vi "Remove Device.vi"(8 "error in (no error)":errorcluster, 11 "Configuration Editor in":refnum<class "Configuration Editor.lvclass">) -> (0 "error out":errorcluster, 3 "Configuration Editor out":refnum<class "Configuration Editor.lvclass">)   [LabVIEW 2023, in "Configuration Editor.lvlib" / "Configuration Editor.lvclass"]
uses:
  Library/Configuration Editor.lvclass
  Library/Configuration Editor.lvclass/Configuration Editor.ctl
  builds/Framework/Configuration.lvlibp/Library/Configuration.lvclass
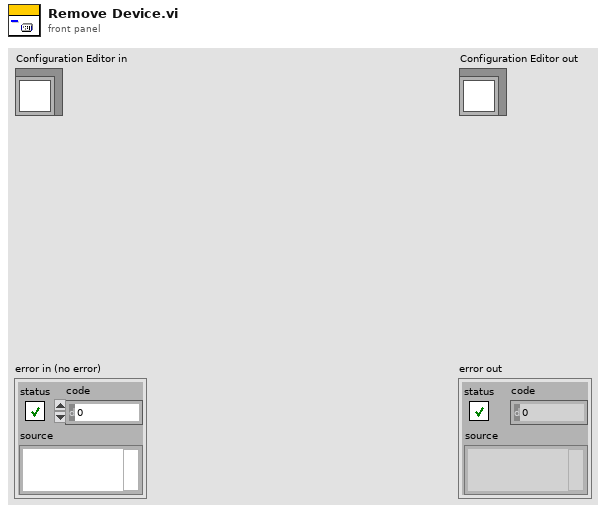
[diagram p1: front panel]
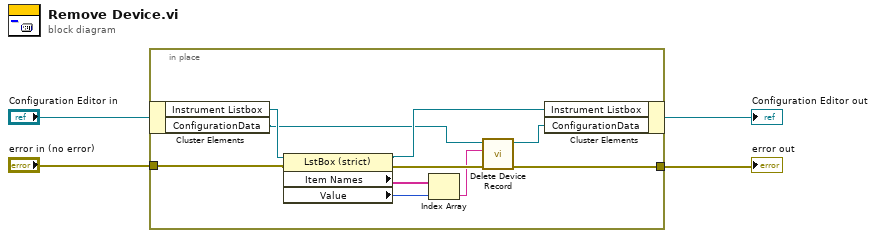
[diagram p0: block diagram]
diagram:
  n1 = in-place {
    in-place-border: "error in (no error)" -> [w11]
    in-place-border: [w6] -> w1
    n2 = in-place-cluster #1("Configuration Editor in") -> ("Instrument Listbox"=w12:refnum<vi>, "ConfigurationData"=w8:refnum<class "Configuration.lvclass">)
    n3 = property class="LstBox (strict)"(reference=w12, error in=w11) -> (reference out=w9:refnum<vi>, error out=w10:errorcluster, "Item Names"=w13:string[], "Value"=w14:i32)
    n4 = Index Array(array=w13, index=w14) -> (element=w5:string)
    n5 = call "Delete Device Record.vi"("error in (no error)"=w10, "Device"=w5, "Configuration in"=w8) -> ("error out"=w6:errorcluster, "Configuration out"=w7:refnum<class "Configuration.lvclass">)  [unwired: 7 in]
    n6 = in-place-cluster #1("Instrument Listbox"=w9, "ConfigurationData"=w7) -> (→"Configuration Editor out":refnum<class "Configuration Editor.lvclass">)
  }
  "error out" <- w1
